vi "measureCapacitanceAndResistance.vi"(8 "error in":errorcluster, 10 "axis":i32, 11 "connection ID in":refnum<k5>) -> (0 "error out":errorcluster, 1 "CapRes":cluster{"capacitance":i32, "resistance":i32}, 2 "axis_out":i32, 3 "connection ID":refnum<k5>)   [LabVIEW 2016]
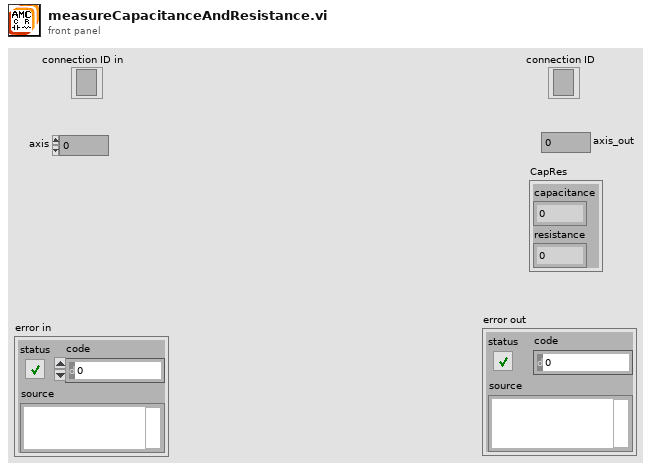
[diagram p1: front panel]
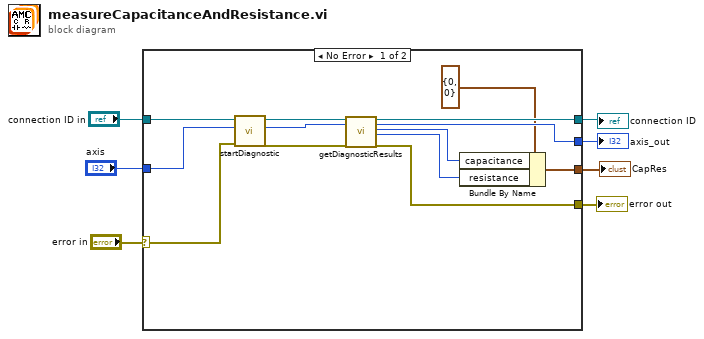
[diagram p0: block diagram]
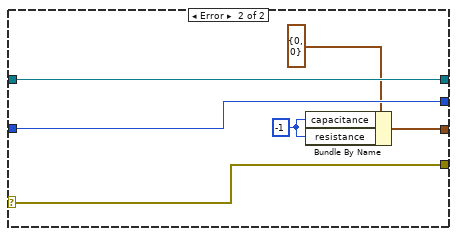
[diagram p2: hidden frame]
diagram:
  n1 = case shown="No Error" "error in" {
    selector: "error in" -> [w14 w24]
    tunnel: "connection ID in" -> [w20 w26]
    tunnel: [w18 w26] -> w6
    tunnel: [w13 w24] -> w5
    tunnel: "axis" -> [w16 w25]
    tunnel: [w12 w25] -> w2
    tunnel: [w8 w21] -> w1
    frame No Error {
      n2 = call "startDiagnostic.vi"("error in"=w14, "axis"=w16, "connection ID"=w20) -> ("error out"=w15:errorcluster, "axis_out"=w17:i32, "connection ID"=w19:refnum<k5>)  [unwired: 6 in]
      n3 = call "getDiagnosticResults.vi"("connection ID"=w19, "axis"=w17, "error in"=w15) -> ("connection ID"=w18:refnum<k5>, "axis_out"=w12:i32, "capacity"=w10:i32, "resistance"=w9:i32, "error out"=w13:errorcluster)  [unwired: 12 in]
      n4 = Bundle By Name(cluster=cluster{"capacitance":i32, "resistance":i32} {"capacitance"=0, "resistance"=0} ("results 2"), "capacitance"=w10, "resistance"=w9) -> (w8:cluster{"capacitance":i32, "resistance":i32})
    }
    frame Error {
      w22 = -1 ("capacity")
      n5 = Bundle By Name(cluster=cluster{"capacitance":i32, "resistance":i32} {"capacitance"=0, "resistance"=0} ("results 2"), "capacitance"=w22, "resistance"=w22) -> (w21:cluster{"capacitance":i32, "resistance":i32})
    }
  }
  "connection ID" <- w6
  "error out" <- w5
  "axis_out" <- w2
  "CapRes" <- w1
